vi "PropertyNodeSample.vi"() -> ()   [LabVIEW 2025]
doc: "Demonstrates a numeric control with the 'Disabled and Grayed Out' state set using a property node; the state can be changed from the front panel and block diagram and then Implements blinking and key focus on a control using a property node; the blinking stops when the user focuses on the input field."
panel:
  in  "stop":bool
  in  "Numeric 4":dbl
  out "Disabled":T1(ring)
  in  "Numeric 3":dbl
  out "Numeric 2":dbl
  in  "Numeric":dbl
  # "Added property node Disabled and grayed out for number, we can change it to enabled or disabled if we want in block diagram"
  # "Added property node Disabled and grayed out for number, we can change it to enabled or disabled if we want in front panel"
  # "Added property node blinking and key focus when when we focus on input it will stop blinking"
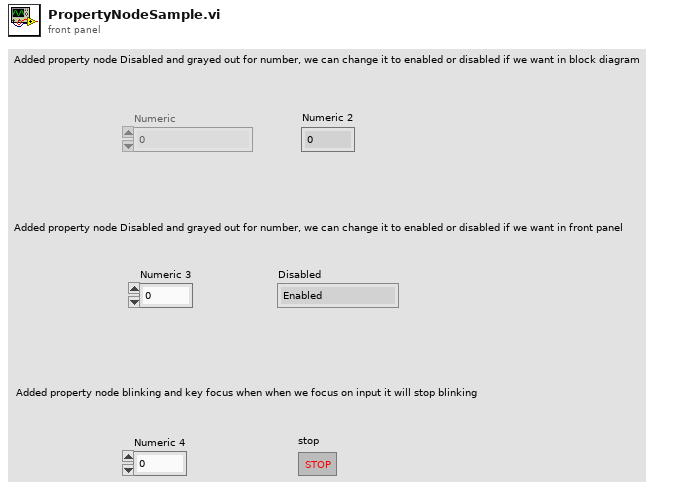
[diagram p1: front panel]
types:
  T1 = enum8{"Enabled", "Disabled", "Disabled and Grayed Out"}
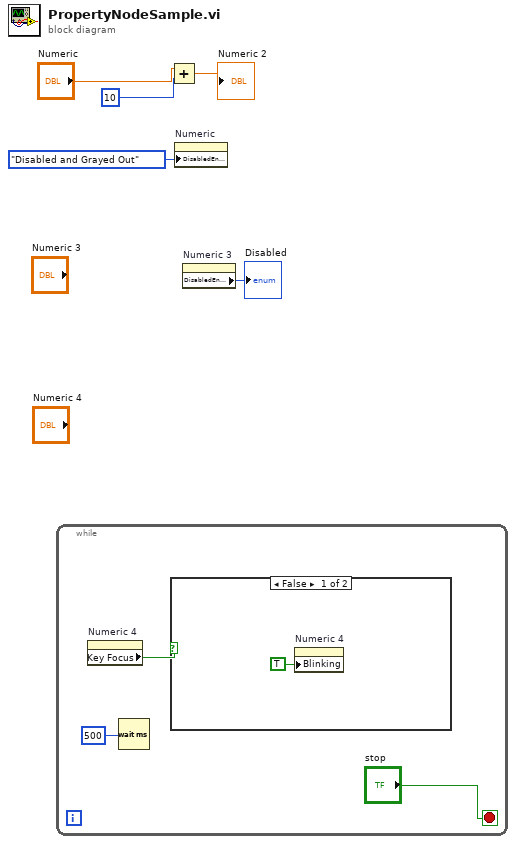
[diagram p0: block diagram]
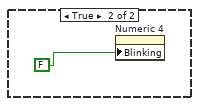
[diagram p2: hidden frame]
diagram:
  n1 = while {
    stop <- "stop" stop-if-true
    n2 = property on="Numeric 4" class="DigNum (strict)"() -> ("Key Focus"=w7:bool)  [unwired: 2 in, 2 out]
    n3 = Wait (ms)(milliseconds to wait=500) -> ()  [unwired: 1 out]
    n4 = case shown="False" w7 {
      frame False {
        n5 = property on="Numeric 4" class="DigNum (strict)"("Blinking"=TRUE) -> ()  [unwired: 2 in, 2 out]
      }
      frame True {
        n6 = property on="Numeric 4" class="DigNum (strict)"("Blinking"=FALSE) -> ()  [unwired: 2 in, 2 out]
      }
    }
  }
  n7 = Add(x="Numeric", y=10) -> (x+y=→"Numeric 2":dbl)
  n8 = property on="Numeric" class="DigNum (strict)"("DisabledEnum"=T1."Disabled and Grayed Out" ("Disabled")) -> ()  [unwired: 2 in, 2 out]
  n9 = property on="Numeric 3" class="DigNum (strict)"() -> ("DisabledEnum"=→"Disabled":T1)  [unwired: 2 in, 2 out]
